vi "2DFilter (SubVI).vi"(0 "Input":u16[][](array[numeric]), 1 "Sample Frequency":dbl, 2 "High cut (Hz)":dbl, 3 "Low cut (Hz)":dbl, 4 "Filter":bool, 5 "Filter type":T1) -> (7 "Filter output":dbl[][](array[numeric]))   [LabVIEW 2016]
uses:
  <vilib>/Analysis/3filter.llb/Filter Passband Type.ctl
  <vilib>/Analysis/3filter.llb/Butterworth Filter (DBL).vi
  <vilib>/Analysis/NI_AALBase.lvlib
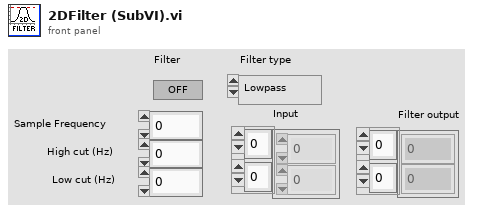
[diagram p1: front panel]
types:
  T1 = typedef "NI_AALBase.lvlib/Filter Passband Type.ctl" = enum32{"Lowpass", "Highpass", "Bandpass", "Bandstop"}
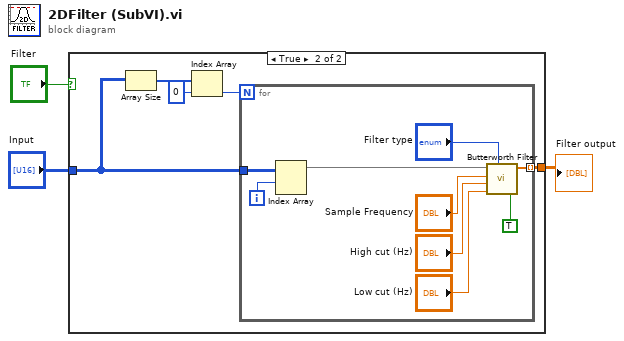
[diagram p0: block diagram]
diagram:
  n1 = case shown="True" "Filter" {
    tunnel: "Input" -> [w4 w7]
    tunnel: [w4 w5] -> w1
    frame False {
    }
    frame True {
      n2 = Array Size(array=w7) -> (size(s)=w9:i32[])
      n3 = Index Array(array=w9, index=0) -> (element=w6:i32)
      n4 = for {
        N: w6 -> [_]
        tunnel: w7 -> [w17]
        tunnel: [w10] -> w5 mode=indexing
        i -> [w16]
        n5 = Index Array(array=w17, index (row)=w16) -> (element=w15:u16[])  [unwired: 1 in]
        n6 = call-poly <vilib>:"Butterworth Filter.vi"("init/cont (init:F)"=TRUE, "filter type"="Filter type", "low cutoff freq: fl"="Low cut (Hz)", "high cutoff freq: fh"="High cut (Hz)", "sampling freq: fs"="Sample Frequency", "X"=w15) -> ("Filtered X"=w10:dbl[])  [unwired: 2 in, 1 out]
      }
    }
  }
  "Filter output" <- w1
